vi "Simple Linear Movement.vi"() -> (1 "stop 2":bool)   [LabVIEW 2012]
uses:
  Global_var.vi
  <userlib>/dhd_sdk7/dhd_sdk7.lvlib
panel:
  out "ID":u8
  in  "Z":dbl min=-0.2 max=0.2 step=0.01
  in  "Y":dbl min=-0.2 max=0.2 step=0.01
  in  "X":dbl min=-0.2 max=0.2 step=0.01
  out "Correct?":bool
  out "flag":bool
  out "Fz":dbl format="%#_3g"
  out "error out":errorcluster
  in  "Start?":bool
  out "Fx":dbl format="%#_3g"
  out "Fy":dbl format="%#_3g"
  in  "stop":bool
  out "Canvas":picture
  # "Delta robot kinetics information"
  # "User Inputs"
  # "Note that real-time updates on the control units (e.g. numeric, string) on the GUI will increase loop delay and as a result robot can become jerky."
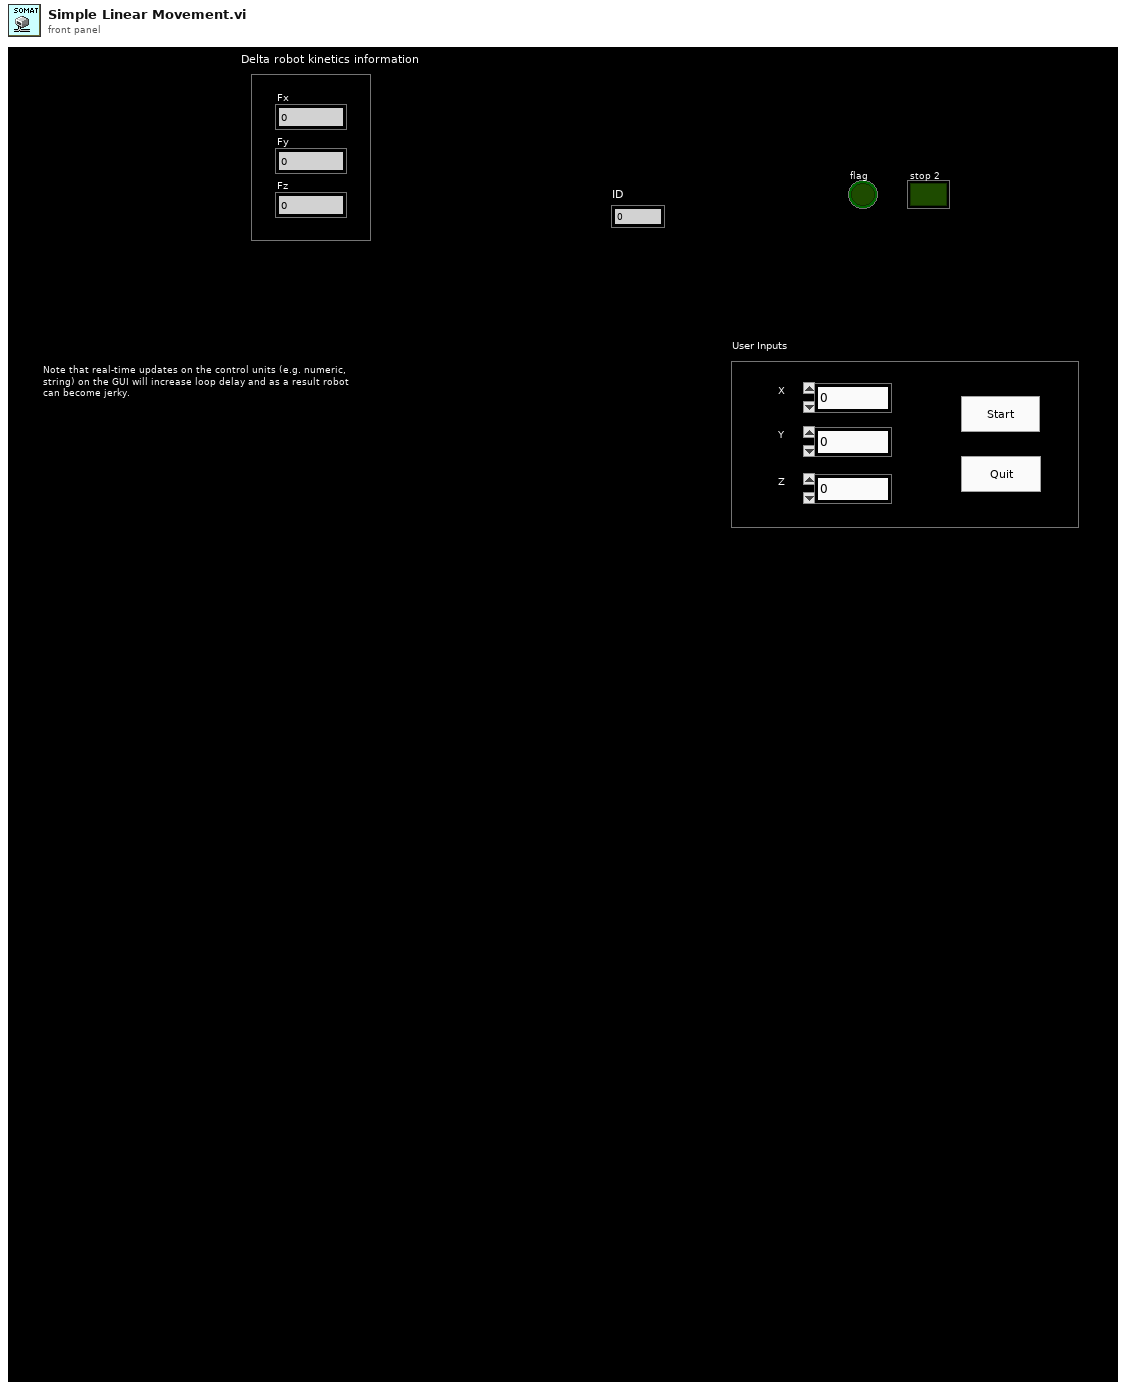
[diagram p1: front panel]
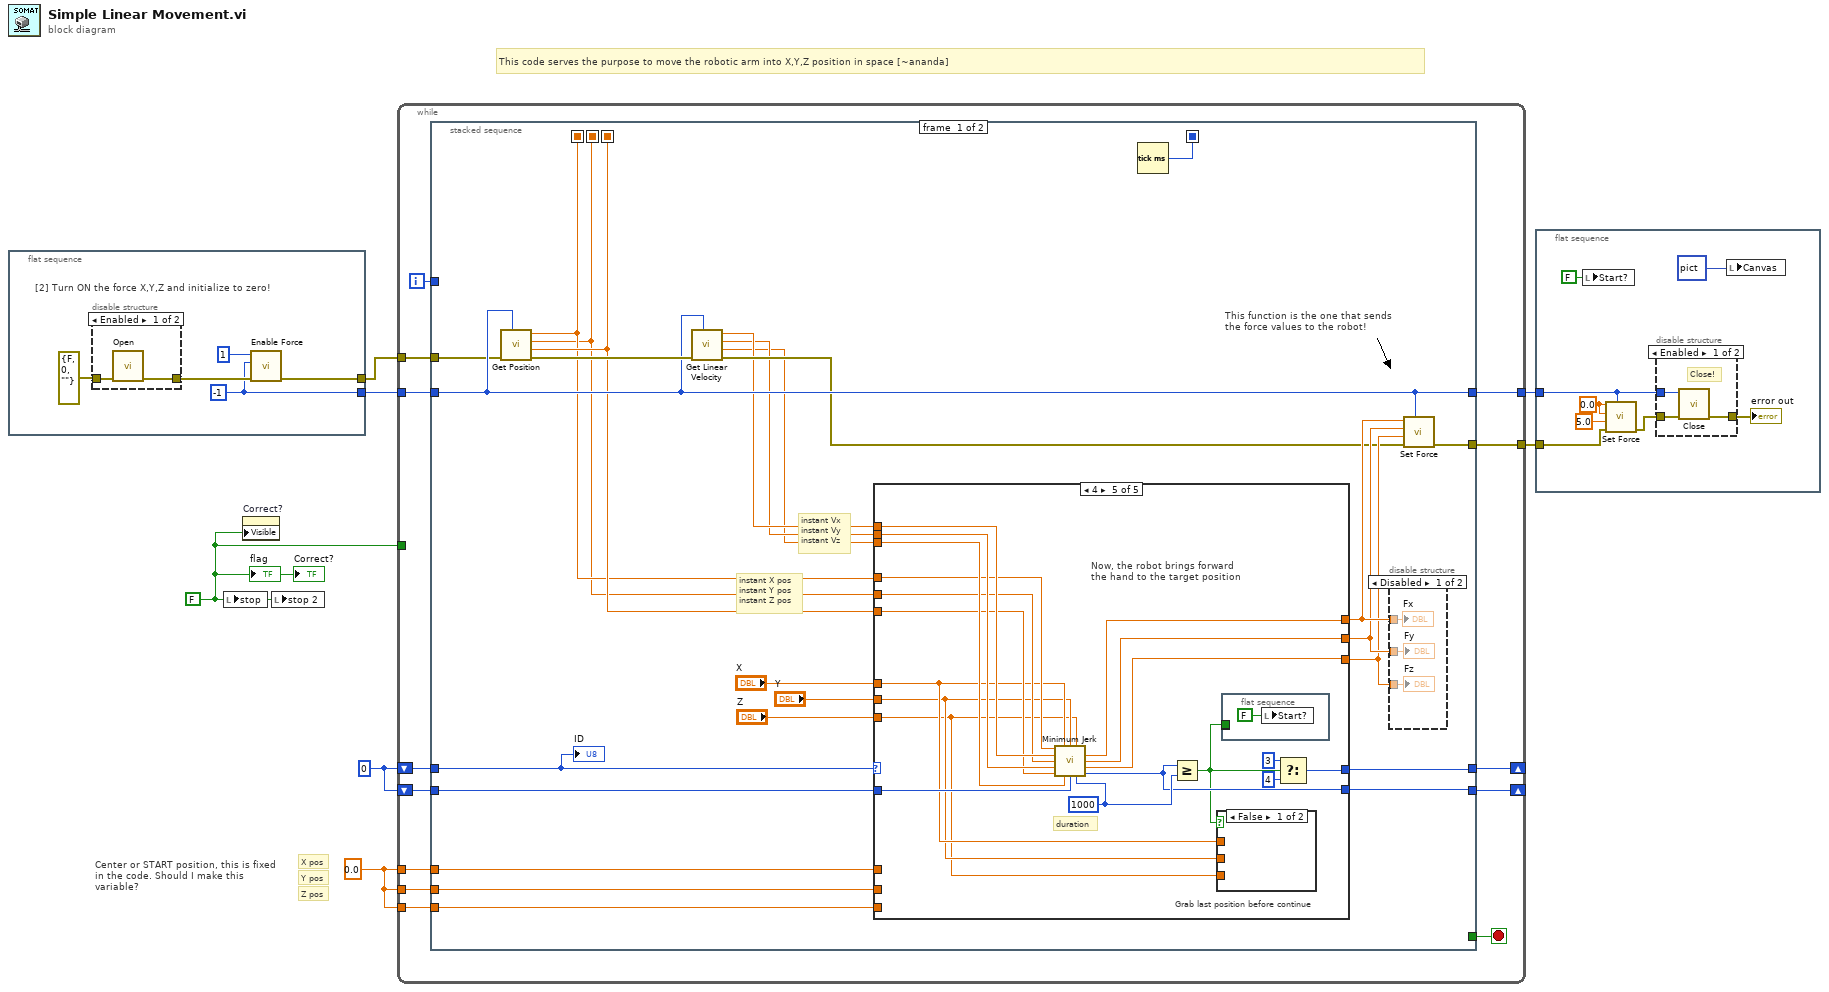
[diagram p0: block diagram]
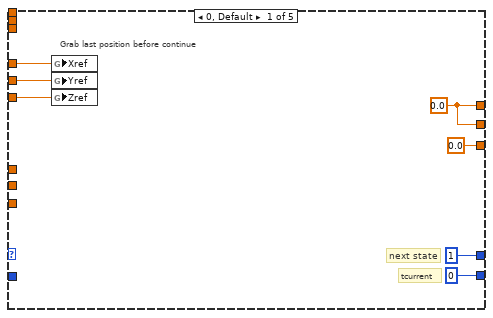
[diagram p3: hidden frame]
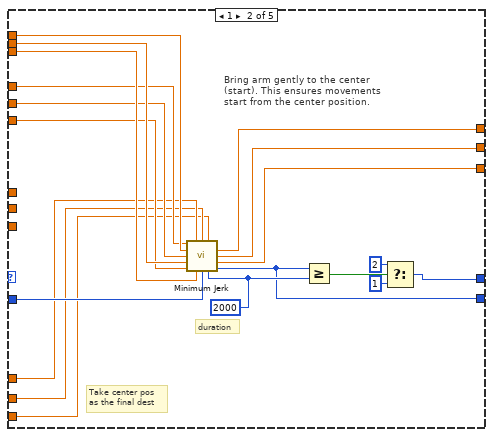
[diagram p4: hidden frame]
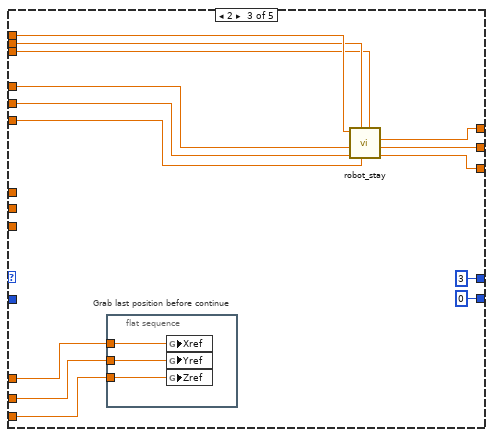
[diagram p5: hidden frame]
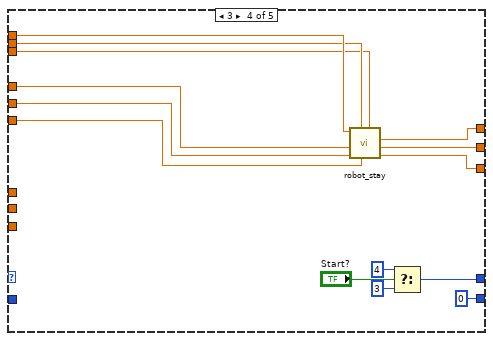
[diagram p6: hidden frame]
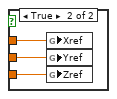
[diagram p7: hidden frame]
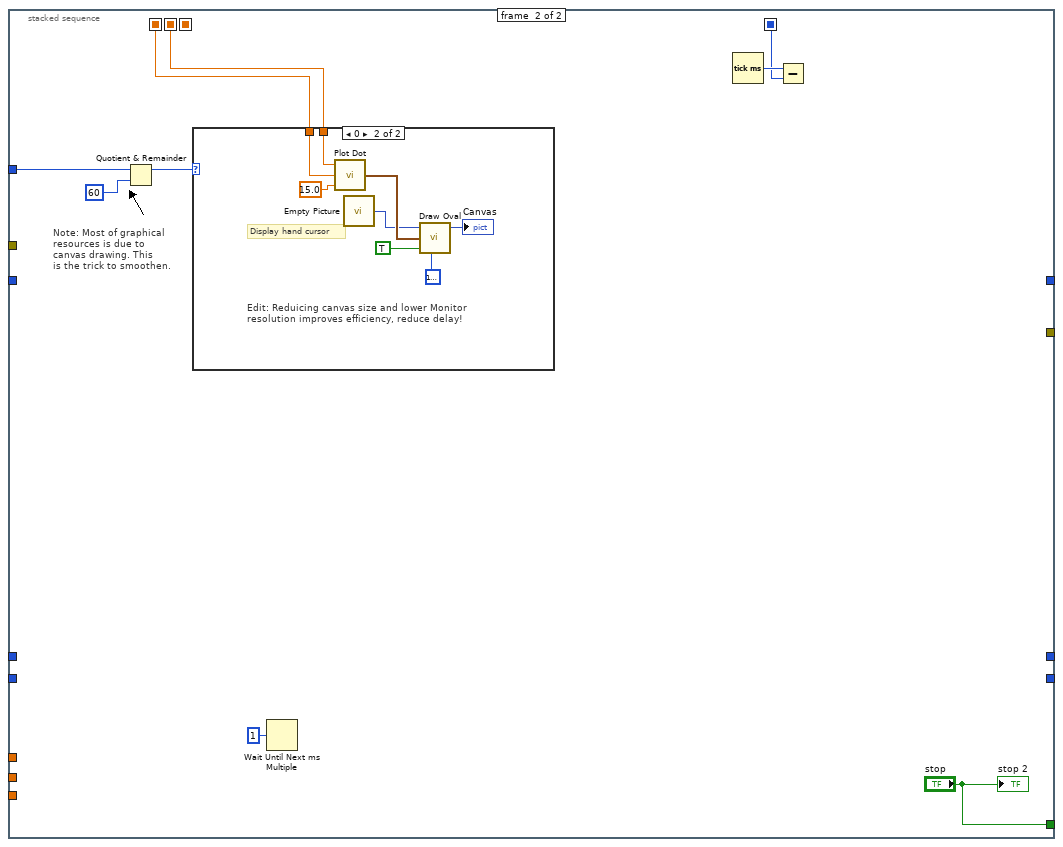
[diagram p8: hidden frame]
diagram:
  w2 = FALSE ("stop")
  w1 = 0.0 ("t")
  w4 = u16 0 ("ID")
  # "This code serves the purpose to move the robotic arm into X,Y,Z position in space [~ananda]"
  # "Z pos"
  # "Y pos"
  # "X pos"
  # "Center or START position, this is fixed in the code. Should I make this variable?"
  n1 = flat-sequence {
    tunnel: [w8] -> w6
    tunnel: [w9] -> w5
    frame #0 {
      w9 = i8 -1 ("ID")
      # "[2] Turn ON the force X,Y,Z and initialize to zero!"
      n2 = disable-structure shown="Enabled" {
        disable-tunnel: errorcluster {"status"=FALSE, "code"=0, "source"=""} ("error out") -> [w14 _]
        disable-tunnel: [w13 _] -> w10
        frame Enabled {
          n3 = call <userlib>:"Open.vi"("error in (no error)"=w14) -> ("error out"=w13:errorcluster)  [unwired: 9 in, 1 out]
        }
        frame Disabled {
        }
      }
      n4 = call <userlib>:"Enable Force.vi"("error in (no error)"=w10, "ID"=w9, "val"=u8 1) -> ("error out"=w8:errorcluster)  [unwired: 7 in, 1 out]
    }
  }
  n5 = local write "stop"(w2) -> ()
  n6 = property on="Correct?" class="Bool (strict)"("Visible"=w2) -> ()  [unwired: 2 in, 2 out]
  n7 = local write "stop 2"(w2) -> ()
  n8 = while {
    tunnel: w5 -> [w26]
    shift-right: [w27] -> _
    shift-left: w4 -> [w24]
    tunnel: [w22] -> w7
    tunnel: w6 -> [w21]
    shift-right: [w19] -> _
    shift-left: w4 -> [w20]
    tunnel: w2 -> [_]
    tunnel: [w18] -> w3
    tunnel: w1 -> [w17]
    tunnel: w1 -> [w16]
    tunnel: w1 -> [w15]
    i -> [w23]
    stop <- w25 stop-if-true
    n9 = stacked-sequence {
      seq-local: [w39 _] -> [_ _]
      seq-local: [w33 _] -> [_ w138]
      seq-local: [w34 _] -> [_ w137]
      seq-local: [w42 _] -> [_ w142]
      tunnel: [w51 _] -> w27
      tunnel: w26 -> [w43 _]
      tunnel: [_ "stop"] -> w25
      tunnel: w24 -> [w52 _]
      tunnel: w23 -> [_ w144]
      tunnel: [w43 _] -> w22
      tunnel: w21 -> [w41 _]
      tunnel: w20 -> [w50 _]
      tunnel: [w49 _] -> w19
      tunnel: [w48 _] -> w18
      tunnel: w17 -> [w30 _]
      tunnel: w16 -> [w29 _]
      tunnel: w15 -> [w28 _]
      frame #0 {
        # "This function is the one that sends \nthe force values to the robot!"
        # "instant Vx\ninstant Vy\ninstant Vz"
        # "instant X pos\ninstant Y pos\ninstant Z pos"
        n10 = call <userlib>:"Get Position.vi"("ID"=w43, "error in (no error)"=w41) -> ("error out"=w44:errorcluster, "pz out"=w39:dbl, "py out"=w33:dbl, "px out"=w34:dbl)  [unwired: 5 in, 1 out]
        n11 = call <userlib>:"Get Linear Velocity.vi"("ID"=w43, "error in (no error)"=w44) -> ("error out"=w40:errorcluster, "vz out"=w36:dbl, "vy out"=w37:dbl, "vx out"=w38:dbl)  [unwired: 5 in, 1 out]
        n12 = case shown="4" w52 {
          tunnel: [u8 1 ("f") w75 u8 3 ("f") w107 w117] -> w51
          tunnel: [w61 w78 w95 w112 w121] -> w47
          tunnel: [w61 w77 w94 w111 w120] -> w46
          tunnel: w50 -> [_ w70 _ _ w122]
          tunnel: [u16 0 ("tcurrent") w74 u32 0 ("millisecond timer value") u32 0 ("millisecond timer value") w118] -> w49
          tunnel: [0.0 ("Fx") w76 w93 w110 w119] -> w45
          tunnel: w34 -> [w58 w69 w88 w102 w125]
          tunnel: w33 -> [w57 w68 w87 w101 w124]
          tunnel: w39 -> [w56 w67 w86 w100 w123]
          tunnel: w38 -> [_ w73 w91 w105 w128]
          tunnel: w37 -> [_ w72 w90 w104 w127]
          tunnel: w36 -> [_ w71 w89 w103 w126]
          tunnel: "X" -> [_ _ _ _ w115]
          tunnel: "Y" -> [_ _ _ _ w114]
          tunnel: "Z" -> [_ _ _ _ w113]
          tunnel: w30 -> [_ w65 w84 _ _]
          tunnel: w29 -> [_ w64 w83 _ _]
          tunnel: w28 -> [_ w63 w82 _ _]
          frame 0, Default {
            w61 = 0.0 ("Fx")
            # "next state"
            # "Grab last position before continue"
            # "tcurrent"
            n13 = global write "Global_var.vi" "Xref"(w58) -> ()
            n14 = global write "Global_var.vi" "Yref"(w57) -> ()
            n15 = global write "Global_var.vi" "Zref"(w56) -> ()
          }
          frame 1 {
            w81 = u16 2000 ("duration")
            # "Take center pos\nas the final dest"
            # "Bring arm gently to the center\n(start). This ensures movements\nstart from the center position."
            # "duration"
            n16 = call "Minimum Jerk.vi"("X"=w69, "Xfinal"=w65, "Yfinal"=w64, "Zfinal"=w63, "Vx"=w73, "Y"=w68, "Vy"=w72, "Z"=w67, "Vz"=w71, "current_n"=w70, "duration"=w81) -> ("Fx"=w78:dbl, "Fy"=w77:dbl, "Fz"=w76:dbl, "n out"=w74:u16)  [unwired: 1 out]
            n17 = Greater Or Equal?(x=w74, y=w81) -> (x >= y?=w66:bool)
            n18 = Select(t=u8 2 ("ID"), s=w66, f=u8 1) -> (s? t:f=w75:u8)
          }
          frame 2 {
            # "Grab last position before continue"
            n19 = flat-sequence {
              tunnel: w84 -> [w98]
              tunnel: w83 -> [w97]
              tunnel: w82 -> [w96]
              frame #0 {
                n20 = global write "Global_var.vi" "Xref"(w98) -> ()
                n21 = global write "Global_var.vi" "Yref"(w97) -> ()
                n22 = global write "Global_var.vi" "Zref"(w96) -> ()
              }
            }
            n23 = call "robot_stay.vi"("Vz"=w89, "Z"=w86, "Vy"=w90, "Y"=w87, "X"=w88, "Vx"=w91) -> ("Fz"=w93:dbl, "Fy"=w94:dbl, "Fx"=w95:dbl)  [unwired: 3 in]
          }
          frame 3 {
            n24 = call "robot_stay.vi"("Vz"=w103, "Z"=w100, "Vy"=w104, "Y"=w101, "X"=w102, "Vx"=w105) -> ("Fz"=w110:dbl, "Fy"=w111:dbl, "Fx"=w112:dbl)  [unwired: 3 in]
            n25 = Select(t=u8 4, s="Start?", f=u8 3) -> (s? t:f=w107:u8)
          }
          frame 4 {
            w131 = u16 1000 ("duration")
            # "Grab last position before continue"
            # "duration"
            # "Now, the robot brings forward\nthe hand to the target position"
            n26 = call "Minimum Jerk.vi"("X"=w125, "Xfinal"=w115, "Yfinal"=w114, "Zfinal"=w113, "Vx"=w128, "Y"=w124, "Vy"=w127, "Z"=w123, "Vz"=w126, "current_n"=w122, "duration"=w131) -> ("Fx"=w121:dbl, "Fy"=w120:dbl, "Fz"=w119:dbl, "n out"=w118:u16)  [unwired: 1 out]
            n27 = Greater Or Equal?(x=w118, y=w131) -> (x >= y?=w116:bool)
            n28 = case shown="False" w116 {
              tunnel: w115 -> [_ w134]
              tunnel: w114 -> [_ w133]
              tunnel: w113 -> [_ w132]
              frame False {
              }
              frame True {
                n29 = global write "Global_var.vi" "Xref"(w134) -> ()
                n30 = global write "Global_var.vi" "Yref"(w133) -> ()
                n31 = global write "Global_var.vi" "Zref"(w132) -> ()
              }
            }
            n32 = flat-sequence {
              tunnel: [w135] -> _
              tunnel: w116 -> [w135]
              frame #0 {
                n33 = local write "Start?"(FALSE ("Start?")) -> ()
              }
            }
            n34 = Select(t=u8 3 ("ID"), s=w116, f=u8 4) -> (s? t:f=w117:u8)
          }
        }
        n35 = Tick Count (ms)() -> (millisecond timer value=w42:u32)
        n36 = disable-structure shown="Disabled" {
          disable-tunnel: w47 -> [w55 _]
          disable-tunnel: w46 -> [w54 _]
          disable-tunnel: w45 -> [w53 _]
          frame Disabled {
            "Fy" <- w54
            "Fx" <- w55
            "Fz" <- w53
          }
          frame Enabled {
          }
        }
        n37 = call <userlib>:"Set Force.vi"("ID"=w43, "error in (no error)"=w40, "fz"=w45, "fy"=w46, "fx"=w47) -> ("error out"=w48:errorcluster)  [unwired: 5 in, 1 out]
        "ID" <- w52
      }
      frame #1 {
        # "Note: Most of graphical resources is due to canvas drawing. This\nis the trick to smoothen."
        n38 = Quotient & Remainder(x=w144, y=60) -> (x-y*floor(x/y)=w140:i32)  [unwired: 1 out]
        n39 = case shown="0" w140 {
          tunnel: w137 -> [_ w147]
          tunnel: w138 -> [_ w148]
          frame 1, Default {
          }
          frame 0 {
            # "Edit: Reduicing canvas size and lower Monitor resolution improves efficiency, reduce delay!"
            # "Display hand cursor"
            n40 = call "Plot Dot.vi"("Diameter"=15.0 ("Size"), "Y"=w147, "X"=w148) -> ("Cluster"=w149:cluster{dbl, dbl, dbl, dbl})
            n41 = call "Empty Picture"() -> ("empty picture"=w146:picture)
            n42 = call <vilib>:"Draw Oval.vi"("picture"=w146, "rect"=w149, "fill?(F)"=TRUE, "color(black)"=u32 16777226) -> ("new picture"=→"Canvas":picture)  [unwired: 5 in]
          }
        }
        n43 = Wait Until Next ms Multiple(millisecond multiple=u32 1) -> ()  [unwired: 1 out]
        n44 = Tick Count (ms)() -> (millisecond timer value=w143:u32)
        n45 = Subtract(x=w143, y=w142) -> ()  [unwired: 1 out]
        "stop 2" <- "stop"
      }
    }
  }
  n46 = flat-sequence {
    tunnel: w7 -> [w161]
    tunnel: w3 -> [w159]
    frame #0 {
      w155 = 0.0 ("fx")
      n47 = local write "Start?"(FALSE ("start")) -> ()
      n48 = call <userlib>:"Set Force.vi"("ID"=w161, "error in (no error)"=w159, "fz"=5.0, "fy"=w155, "fx"=w155) -> ("error out"=w160:errorcluster)  [unwired: 5 in, 1 out]
      n49 = disable-structure shown="Enabled" {
        disable-tunnel: w161 -> [w164 _]
        disable-tunnel: w160 -> [w163 w165]
        disable-tunnel: [w162 w165] -> w154
        frame Enabled {
          # "Close!"
          n50 = call <userlib>:"Close.vi"("error in (no error)"=w163, "ID"=w164) -> ("error out"=w162:errorcluster)  [unwired: 8 in, 1 out]
        }
        frame Disabled {
        }
      }
      "error out" <- w154
      n51 = local write "Canvas"(picture data[5B] ("Canvas")) -> ()
    }
  }
  "flag" <- w2
  "Correct?" <- w2
